vi "Run.vi"(8 "error in (no error)":errorcluster, 11 "App in":refnum<class "App.lvclass">) -> (0 "error out":errorcluster, 3 "App out":refnum<class "App.lvclass">)   [LabVIEW 2020, in "PicoG-App.lvlib" / "App.lvclass"]
uses:
  App.lvclass
  App.lvclass/App.ctl
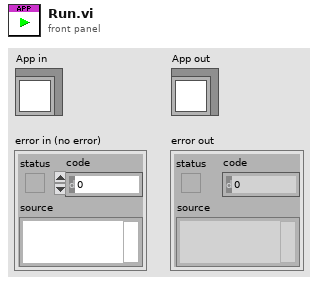
[diagram p1: front panel]
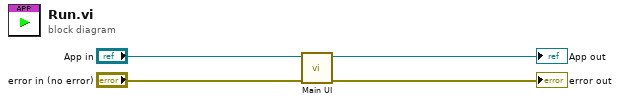
[diagram p0: block diagram]
diagram:
  n1 = call "Main UI.vi"("error in (no error)"="error in (no error)", "App in"="App in") -> ("error out"=→"error out":errorcluster, "App out"=→"App out":refnum<class "App.lvclass">)  [unwired: 8 in]
